vi "KeithleyClose.vi"(8 "Keithley Error In":errorcluster, 10 "Node In":string, 11 "KeithleyVISA In":refnum<visa-resource-name>) -> (0 "Heater Error":errorcluster={"status"=FALSE, "code"=1073676293, "source"="VISA Read in Keithley 2600 Series.lvlib:Print Number.vi->Keithley 2600 Series.lvlib:Measure.vi->Turbulence.vi"})   [LabVIEW 2018]
uses:
  <instrlib>/Keithley 2600 Series/Public/Channel.ctl
  <instrlib>/Keithley 2600 Series/Keithley 2600 Series.lvlib
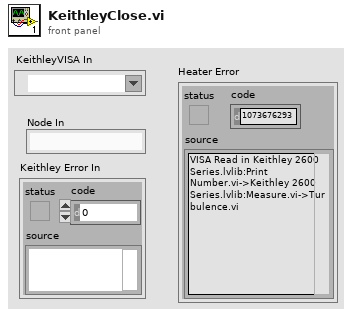
[diagram p1: front panel]
types:
  T1 = typedef "Keithley 2600 Series.lvlib/Channel.ctl" = enum32{"Channel A", "Channel B"}
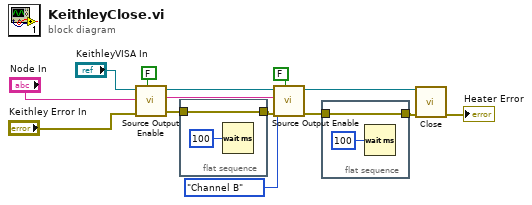
[diagram p0: block diagram]
diagram:
  n1 = call <instrlib>:"Source Output Enable.vi"("Output (Off)"=FALSE, "error in (no error)"="Keithley Error In", "Node In"="Node In", "VISA resource name"="KeithleyVISA In") -> ("error out"=w9:errorcluster, "Node Out"=w7:string, "VISA resource name out"=w8:refnum<visa-resource-name>)  [unwired: 4 in, 1 out]
  n2 = flat-sequence {
    tunnel: w9 -> [w15]
    tunnel: [w15] -> w10
    frame #0 {
      n3 = Wait (ms)(milliseconds to wait=u32 100) -> ()  [unwired: 1 out]
    }
  }
  n4 = call <instrlib>:"Source Output Enable.vi"("Output (Off)"=FALSE, "error in (no error)"=w10, "Channel (Channel A)"=Channel."Channel B", "Node In"=w7, "VISA resource name"=w8) -> ("error out"=w13:errorcluster, "VISA resource name out"=w11:refnum<visa-resource-name>)  [unwired: 3 in, 2 out]
  n5 = flat-sequence {
    tunnel: w13 -> [w17]
    tunnel: [w17] -> w12
    frame #0 {
      n6 = Wait (ms)(milliseconds to wait=u32 100) -> ()  [unwired: 1 out]
    }
  }
  n7 = call <instrlib>:"Close.vi"("error in (no error)"=w12, "VISA resource name"=w11) -> ("error out"=→"Heater Error":errorcluster)  [unwired: 9 in]
